vi "Initialize UI.vi"(8 "error in":errorcluster, 11 "BigMAQ in":refnum<class "BigMAQ.lvclass">) -> (0 "error out":errorcluster, 3 "BigMAQ out":refnum<class "BigMAQ.lvclass">)   [LabVIEW 2019, in "BigMAQ.lvclass"]
uses:
  BigMAQ.lvclass
  BigMAQ.lvclass/BigMAQ.ctl
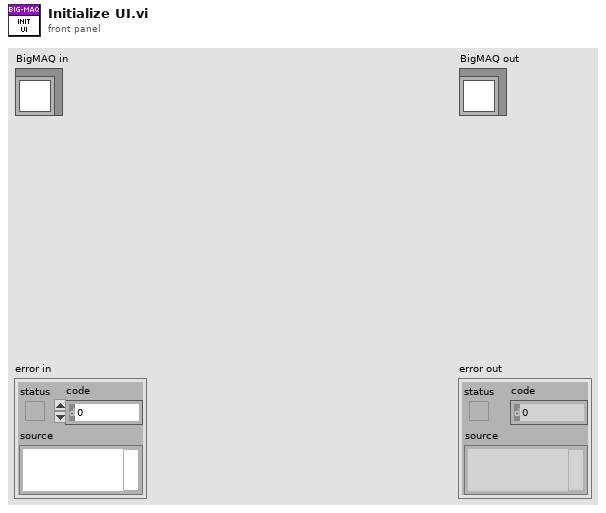
[diagram p1: front panel]
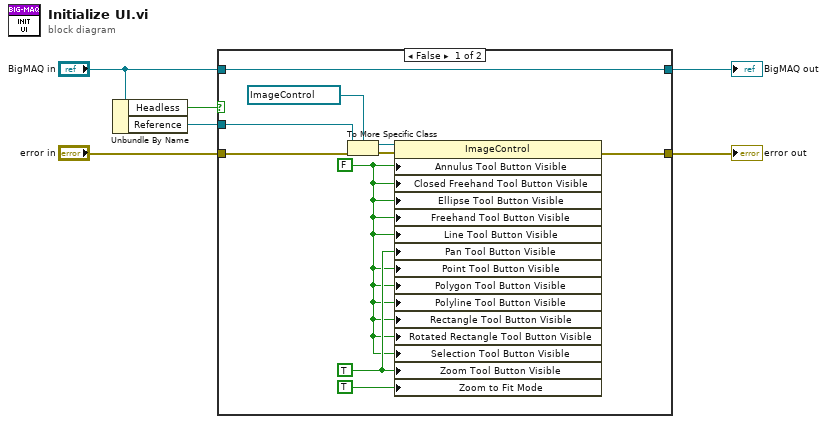
[diagram p0: block diagram]
diagram:
  n1 = Unbundle By Name("BigMAQ in") -> ("Headless"=w3:bool, "Reference"=w6:refnum<vi>)
  n2 = case shown="False" w3 {
    tunnel: w6 -> [w11 _]
    tunnel: "error in" -> [w8 w18]
    tunnel: [w14 w18] -> w4
    tunnel: "BigMAQ in" -> [w12 w17]
    tunnel: [w12 w17] -> w1
    frame False {
      w13 = FALSE
      w16 = TRUE
      n3 = To More Specific Class(target class=refnum<vi> refnum ("reference"), reference=w11, error in=w8) -> (specific class reference=w9:refnum<vi>, error out=w7:errorcluster)
      n4 = property on="Property Node" class="ImageControl"(reference=w9, error in=w7, "Annulus Tool Button Visible"=w13, "Closed Freehand Tool Button Visible"=w13, "Ellipse Tool Button Visible"=w13, "Freehand Tool Button Visible"=w13, "Line Tool Button Visible"=w13, "Pan Tool Button Visible"=w16, "Point Tool Button Visible"=w13, "Polygon Tool Button Visible"=w13, "Polyline Tool Button Visible"=w13, "Rectangle Tool Button Visible"=w13, "Rotated Rectangle Tool Button Visible"=w13, "Selection Tool Button Visible"=w13, "Zoom Tool Button Visible"=w16, "Zoom to Fit Mode"=TRUE) -> (error out=w14:errorcluster)  [unwired: 1 out]
    }
    frame True {
    }
  }
  "error out" <- w4
  "BigMAQ out" <- w1
